vi "Get Stop Status.vi"(8 "error in (no error)":errorcluster, 11 "Teststand in":refnum<class "Teststand.lvclass">) -> (0 "error out":errorcluster, 2 "Value":bool, 3 "Teststand out":refnum<class "Teststand.lvclass">)   [LabVIEW 2023, in "HardwareAbstractionLayer_LVOOP.lvlib" / "Teststand.lvclass"]
uses:
  Teststand.lvclass
  Teststand.lvclass/Teststand.ctl
  <vilib>/addons/TestStand/_TSUtility.llb/TestStand - Get Property Value (Boolean).vi
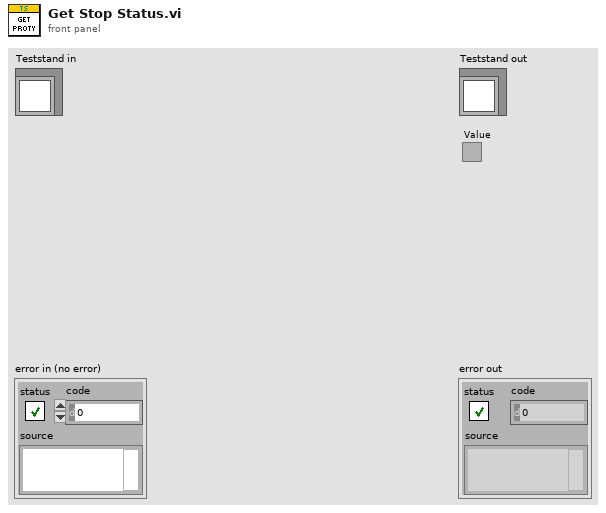
[diagram p1: front panel]
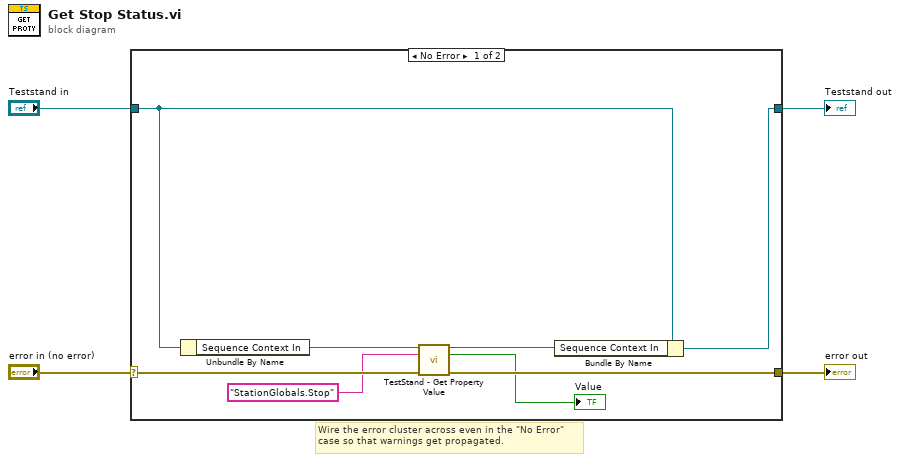
[diagram p0: block diagram]
diagram:
  # "Wire the error cluster across even in the \"No Error\"\ncase so that warnings get propagated."
  n1 = case shown="No Error" "error in (no error)" {
    selector: "error in (no error)" -> [w12 w14]
    tunnel: [w11 w14] -> w3
    tunnel: [w8 w13] -> w1
    tunnel: "Teststand in" -> [w9 w13]
    frame No Error {
      n2 = Unbundle By Name(w9) -> ("Sequence Context In"=w10:refnum<k7>)
      n3 = call-poly <vilib>:"TestStand - Get Property Value.vi"("Sequence Context In"=w10, "Lookup String"="StationGlobals.Stop", "error in (no error)"=w12) -> ("Sequence Context Out"=w7:refnum<k7>, "Value"=→"Value":bool, "error out"=w11:errorcluster)  [unwired: 10 in]
      n4 = Bundle By Name(cluster=w9, "Sequence Context In"=w7) -> (w8:refnum<class "Teststand.lvclass">)
    }
    frame Error {
    }
  }
  "error out" <- w3
  "Teststand out" <- w1
